vi "classify error.vi"(8 "error to classify":errorcluster, 10 "attempt recovery?":bool, 11 "asynchronous execution module runtime In":refnum<class "asynchronous execution module runtime.lvclass">) -> (0 "classified error":errorcluster, 2 "error classification":T1, 3 "asynchronous execution module runtime Out":refnum<class "asynchronous execution module runtime.lvclass">)   [LabVIEW 2013, in "asynchronous execution module runtime.lvclass"]
doc: "Allows a component to classify an error generated at any point during execution. This <b>error classification</b> can then be used by calling code to determine if execution can continue. In addition, this function can be used to allow a component to clear an error, convert an error to a warning, or attempt to recover from an error. Recovery may be attempted only if <b>attempt recovery?</b> is true."
uses:
  asynchronous execution module runtime.lvclass
  <vilib>/NI/Tag Bus Module Framework/runtime/error classification.ctl
  asynchronous execution module runtime.lvclass/asynchronous execution module runtime.ctl
  <vilib>/NI/Tag Bus Module Framework/runtime/TBM module execution interface.lvclass
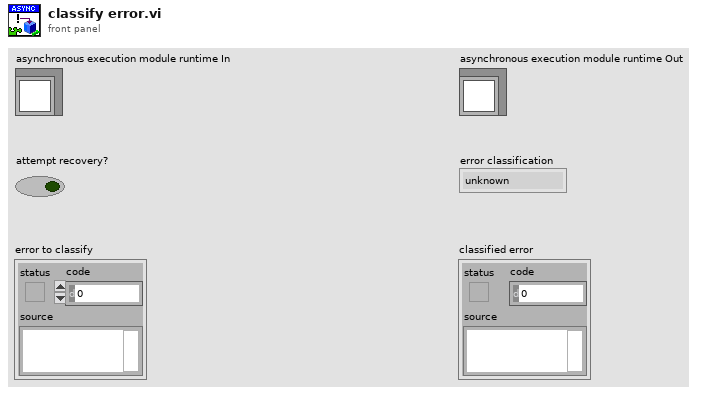
[diagram p1: front panel]
types:
  T1 = typedef "TBM module execution interface.lvclass/error classification.ctl" = enum16{"unknown", "none", "trivial", "recoverable", "critical"}
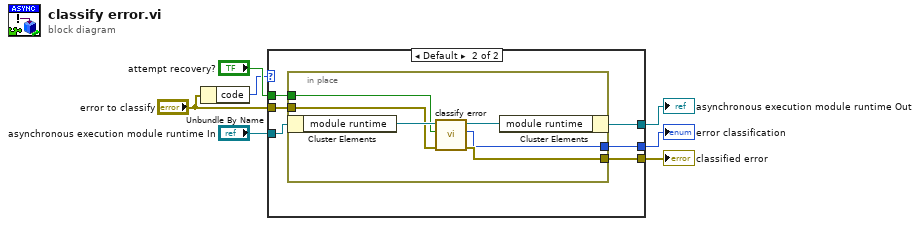
[diagram p0: block diagram]
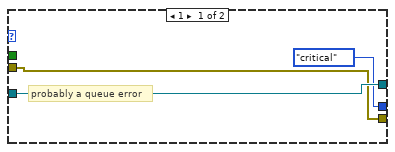
[diagram p2: hidden frame]
diagram:
  n1 = Unbundle By Name("error to classify") -> ("code"=w1:i32)
  n2 = case shown="Default" w1 {
    tunnel: "asynchronous execution module runtime In" -> [w10 w16]
    tunnel: [w10 w15] -> w6
    tunnel: [w8 w14] -> w5
    tunnel: [error_classification."critical" ("error classification") w13] -> w4
    tunnel: "error to classify" -> [w8 w12]
    tunnel: "attempt recovery?" -> [_ w11]
    frame 1 {
      # "probably a queue error"
    }
    frame Default {
      n3 = in-place {
        in-place-border: [w20] -> w14
        in-place-border: [w19] -> w13
        in-place-border: w12 -> [w18]
        in-place-border: w11 -> [w17]
        n4 = in-place-cluster #1(w16) -> ("module runtime"=w22:refnum<class "TBM module execution interface.lvclass">)
        n5 = call-dynamic "classify error.vi"("error to classify"=w18, "attempt recovery?"=w17, "module in"=w22) -> ("classified error"=w20:errorcluster, "error classification"=w19:T1, "module out"=w21:refnum<class "TBM module execution interface.lvclass">)  [unwired: 6 in]
        n6 = in-place-cluster #1("module runtime"=w21) -> (w15:refnum<class "asynchronous execution module runtime.lvclass">)
      }
    }
  }
  "asynchronous execution module runtime Out" <- w6
  "error classification" <- w4
  "classified error" <- w5
